vi "mcapChannelLocator.set.vi"(8 "error in (no error)":errorcluster, 10 "nominal types.lvlib:channelFilter.lvlib:include.lvclass":refnum<class "include.lvclass">, 11 "mcap in":refnum<class "mcap.lvclass">) -> (0 "error out":errorcluster, 3 "mcap out":refnum<class "mcap.lvclass">)   [LabVIEW 2020, in "nominal types.lvlib" / "timestampManifest.lvlib" / "mcap.lvclass"]
uses:
  mcap.lvclass
  mcap.lvclass/mcap.ctl
  include/include.lvclass
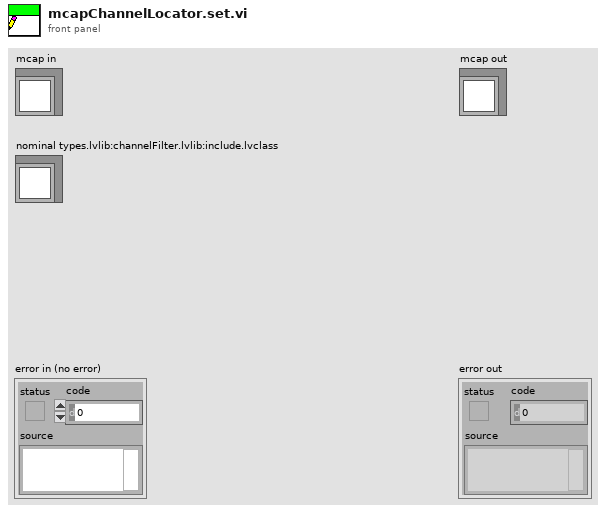
[diagram p1: front panel]
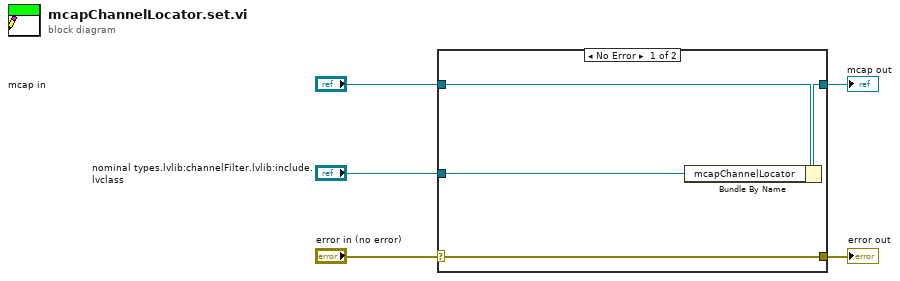
[diagram p0: block diagram]
diagram:
  n1 = case shown="No Error" "error in (no error)" {
    selector: "error in (no error)" -> [w9 w10]
    tunnel: [w9 w10] -> w4
    tunnel: [w7 w11] -> w2
    tunnel: "mcap in" -> [w8 w11]
    tunnel: "nominal types.lvlib:channelFilter.lvlib:include.lvclass" -> [w6 _]
    frame No Error {
      n2 = Bundle By Name(cluster=w8, "mcapChannelLocator"=w6) -> (w7:refnum<class "mcap.lvclass">)
    }
    frame Error {
    }
  }
  "error out" <- w4
  "mcap out" <- w2
